vi "Write Job Description.vi"(10 "Job Description":string, 11 "Build Job in":refnum<class "Build Job.lvclass">) -> (3 "Build Job out":refnum<class "Build Job.lvclass">)   [LabVIEW 2014, in "Build Job.lvclass"]
uses:
  Build Job.lvclass
  Build Job.lvclass/Build Job.ctl
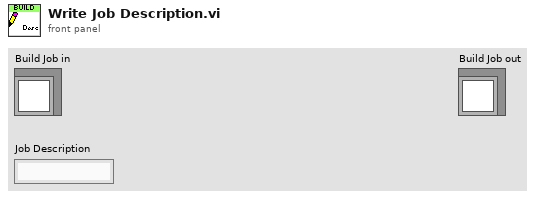
[diagram p1: front panel]
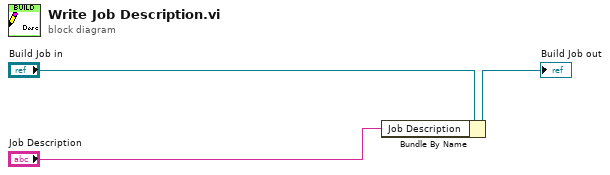
[diagram p0: block diagram]
diagram:
  n1 = Bundle By Name(cluster="Build Job in", "Job Description"="Job Description") -> (→"Build Job out":refnum<class "Build Job.lvclass">)
